vi "uTTA_Send_CalFile.vi"() -> ()   [LabVIEW 2021]
panel:
  out "HPB":u8(slide) scale=0.0..100.0
  out "Progress":string
  out "error out":errorcluster
  in  "Start":bool
  in  "ucf-File":path
  in  "uTTA COM-Port":refnum<visa-resource-name>
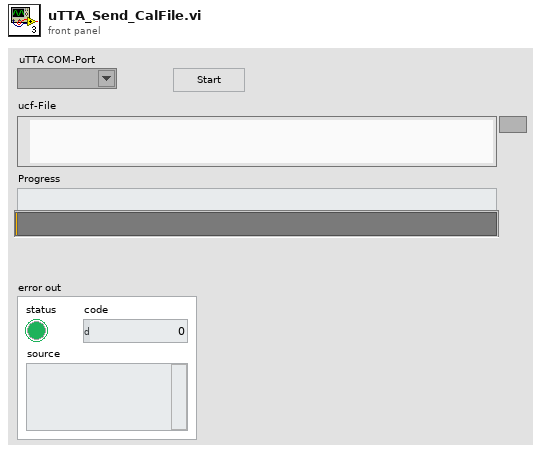
[diagram p1: front panel]
types:
  T1 = enum8{"Enabled", "Disabled", "Disabled and Grayed Out"}
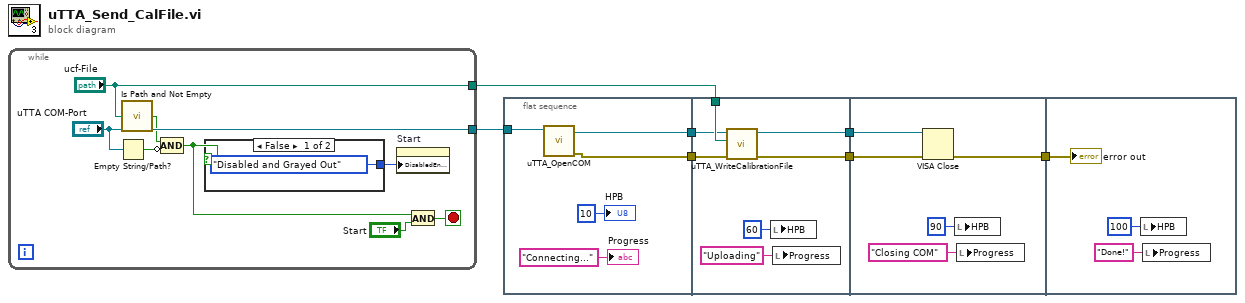
[diagram p0: block diagram]
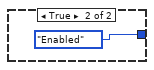
[diagram p2: hidden frame]
diagram:
  n1 = while {
    tunnel: ["uTTA COM-Port"] -> w7
    tunnel: ["ucf-File"] -> w6
    stop <- w8 stop-if-true
    n2 = Empty String/Path?(string/path="uTTA COM-Port") -> (empty?=w12:bool)
    n3 = call <vilib>:"Is Path and Not Empty.vi"("path"="ucf-File") -> ("Is Path and Not Empty?"=w13:bool)  [unwired: 4 in]
    n4 = Compound Arithmetic op=AND(w13, invert w12) -> (w10:bool)
    n5 = case shown="False" w10 {
      tunnel: [T1."Disabled and Grayed Out" ("Disabled") T1."Enabled" ("Disabled")] -> w11
      frame False {
      }
      frame True {
      }
    }
    n6 = property on="Start" class="Bool"("DisabledEnum"=w11) -> ()  [unwired: 2 in, 2 out]
    n7 = And(x=w10, y="Start") -> (x .and. y?=w8:bool)
  }
  n8 = flat-sequence {
    tunnel: w7 -> [w22]
    tunnel: [w21] -> w5
    tunnel: [w20] -> w4
    tunnel: w6 -> [w29]
    tunnel: w5 -> [w28]
    tunnel: w4 -> [w27]
    tunnel: [w24] -> w3
    tunnel: [w23] -> w2
    tunnel: w3 -> [w32]
    tunnel: w2 -> [w31]
    tunnel: [w30] -> w1
    tunnel: w1 -> [w35]
    frame #0 {
      n9 = call "uTTA_OpenCOM.vi"("VISA in"=w22) -> ("error out"=w20:errorcluster, "VISA out"=w21:refnum<visa-resource-name>)  [unwired: 8 in, 1 out]
      "Progress" <- "Connecting..." ("Progress")
      "HPB" <- u8 10 ("HPB")
    }
    frame #1 {
      n10 = call "uTTA_WriteCalibrationFile.vi"("error in"=w27, "ucf-File"=w29, "VISA Refnum in"=w28) -> ("error out"=w23:errorcluster, "VISA Refnum out"=w24:refnum<visa-resource-name>)  [unwired: 2 in, 1 out]
      n11 = local write "HPB"(u8 60 ("HPB")) -> ()
      n12 = local write "Progress"("Uploading" ("Progress")) -> ()
    }
    frame #2 {
      n13 = VISA Close(VISA resource name=w32, error in (no error)=w31) -> (error out=w30:errorcluster)
      n14 = local write "HPB"(u8 90 ("HPB")) -> ()
      n15 = local write "Progress"("Closing COM" ("Progress")) -> ()
    }
    frame #3 {
      n16 = local write "HPB"(u8 100 ("HPB")) -> ()
      n17 = local write "Progress"("Done!" ("Progress")) -> ()
      "error out" <- w35
    }
  }
